vi "WFM MNGR INIT.vi"(8 "error in (no error)":errorcluster, 10 "Sequence File":refnum<k7>, 11 "WFM MNGR in":refnum<class "QPA MSMT Waveform Manager.lvclass">) -> (0 "error out":errorcluster, 3 "WFM MNGR out":refnum<class "QPA MSMT Waveform Manager.lvclass">)   [LabVIEW 2016, in "QPA MSMT Waveform Manager.lvclass"]
uses:
  QPA MSMT Waveform Manager.lvclass
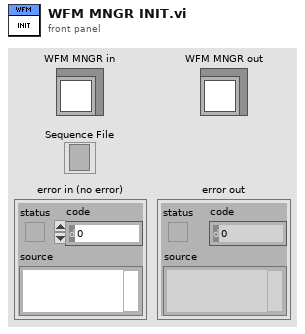
[diagram p1: front panel]
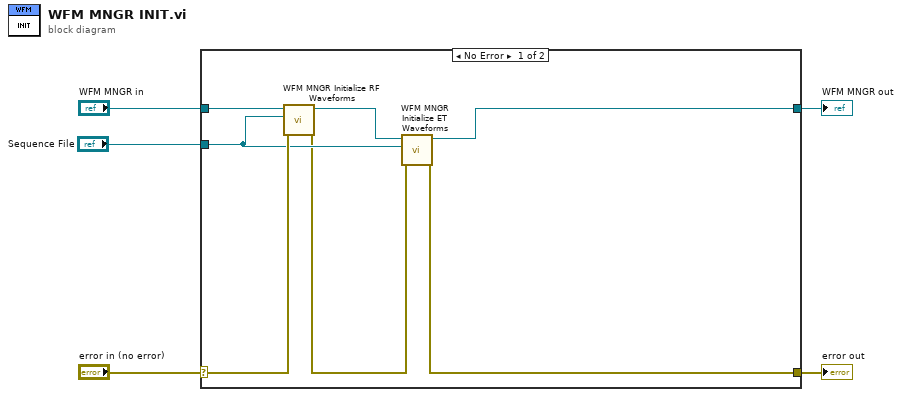
[diagram p0: block diagram]
diagram:
  n1 = case shown="No Error" "error in (no error)" {
    selector: "error in (no error)" -> [w11 w14]
    tunnel: [w6 w14] -> w4
    tunnel: [w8 w13] -> w2
    tunnel: "WFM MNGR in" -> [w12 w13]
    tunnel: "Sequence File" -> [w10 _]
    frame No Error {
      n2 = call "WFM MNGR Initialize RF Waveforms.vi"("error in (no error)"=w11, "Sequence File"=w10, "WFM MNGR in"=w12) -> ("error out"=w7:errorcluster, "WFM MNGR out"=w9:refnum<class "QPA MSMT Waveform Manager.lvclass">)  [unwired: 7 in]
      n3 = call "WFM MNGR Initialize ET Waveforms.vi"("error in (no error)"=w7, "Sequence File"=w10, "WFM MNGR in"=w9) -> ("error out"=w6:errorcluster, "WFM MNGR out"=w8:refnum<class "QPA MSMT Waveform Manager.lvclass">)  [unwired: 7 in]
    }
    frame Error {
    }
  }
  "error out" <- w4
  "WFM MNGR out" <- w2
